vi "S2C_FORNAX_Proc_UpdateGlobals.vi"(8 "Error In":errorcluster, 9 "Values":string[](array[string]), 10 "Keys":string[](array[string]), 11 "Section":string) -> (0 "Error Out":errorcluster)   [LabVIEW 2015]
doc: "Loads setting file values into their respective globals."
uses:
  S2C_FORNAX_Proc_Globals.vi
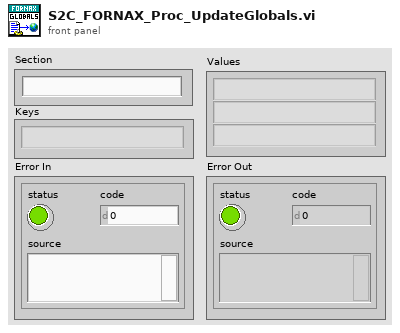
[diagram p1: front panel]
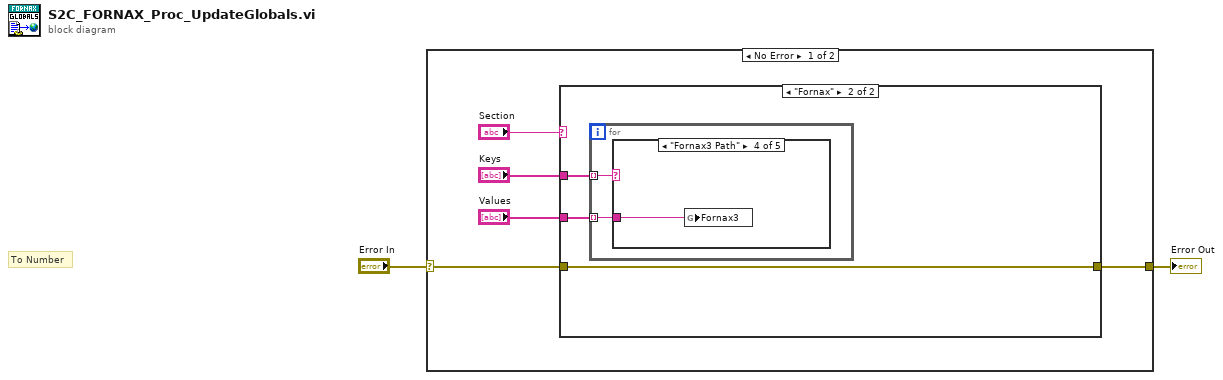
[diagram p0: block diagram]
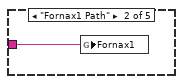
[diagram p4: hidden frame]
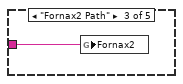
[diagram p5: hidden frame]
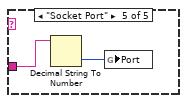
[diagram p6: hidden frame]
diagram:
  # "To Number"
  n1 = case shown="No Error" "Error In" {
    selector: "Error In" -> [w7 w19]
    tunnel: [w3 w19] -> w1
    frame No Error {
      n2 = case shown="\"Fornax\"" "Section" {
        tunnel: "Values" -> [_ w10]
        tunnel: w7 -> [w8 w9]
        tunnel: [w8 w9] -> w3
        tunnel: "Keys" -> [_ w11]
        frame "Other", Default {
        }
        frame "Fornax" {
          n3 = for {
            tunnel: w11 -> [w13] mode=indexing
            tunnel: w10 -> [w12] mode=indexing
            n4 = case shown="\"Fornax3 Path\"" w13 {
              tunnel: w12 -> [_ w14 w15 w16 w18]
              frame "Unknown", Default {
              }
              frame "Fornax1 Path" {
                n5 = global write "S2C_FORNAX_Proc_Globals.vi" "Fornax1"(w14) -> ()
              }
              frame "Fornax2 Path" {
                n6 = global write "S2C_FORNAX_Proc_Globals.vi" "Fornax2"(w15) -> ()
              }
              frame "Fornax3 Path" {
                n7 = global write "S2C_FORNAX_Proc_Globals.vi" "Fornax3"(w16) -> ()
              }
              frame "Socket Port" {
                n8 = Decimal String To Number(string=w18) -> (number=w17:i32)  [unwired: 2 in, 1 out]
                n9 = global write "S2C_FORNAX_Proc_Globals.vi" "Port"(w17) -> ()
              }
            }
          }
        }
      }
    }
    frame Error {
    }
  }
  "Error Out" <- w1
